vi "Periodic Tasks.vi"(8 "error in":errorcluster) -> ()   [LabVIEW 2019]
doc: "This VI runs in parallel to other tasks. It can contain as many user-defined periodic loops as you need. These can carry out PID or other sorts of timed response."
uses:
  <vilib>/Rock Robotics/WPI/ThirdParty/Sensors/navX/_TypeDefs/Flags/Z900_navX_Flags_HardwareRevTypeDef.ctl
  <vilib>/Rock Robotics/WPI/ThirdParty/Sensors/navX/_TypeDefs/Flags/Z900_navX_Flags_OmnimountConfigTypeDef.ctl
  <vilib>/Rock Robotics/WPI/ThirdParty/Sensors/navX/_TypeDefs/Flags/Z900_navX_Flags_OpStatusTypeDef.ctl
  <vilib>/Rock Robotics/WPI/ThirdParty/Sensors/navX/_TypeDefs/Flags/Z900_navX_Flags_CalibrationStatusTypeDef.ctl
  <vilib>/Rock Robotics/WPI/ThirdParty/Sensors/navX/_TypeDefs/Z900_navX_SerialStreamTypeDef.ctl
  <vilib>/Rock Robotics/WPI/ThirdParty/Sensors/navX/_TypeDefs/FRIC_navX_TestStatesTypeDef_I2C.ctl
  <vilib>/Rock Robotics/WPI/ThirdParty/Sensors/navX/_TypeDefs/FRIC_navX_DeviceNumbersTypeDef.ctl
  <vilib>/Rock Robotics/WPI/Utilities/WPI_GetSetVariantRefNum.vi
  <vilib>/Rock Robotics/Network Tables/NT Write Number.vi
  <vilib>/Rock Robotics/Network Tables/NT Read Number.vi
  <vilib>/Rock Robotics/WPI/ThirdParty/Sensors/navX/_Processing Loop/FRIC_navX_Internal_SPI_ProcessingLoop.vi
  <vilib>/Rock Robotics/WPI/ThirdParty/Sensors/navX/_Processing Loop/FRIC_navX_Internal_I2C_ProcessingLoop.vi
  <vilib>/Rock Robotics/WPI/ThirdParty/Sensors/navX/_Processing Loop/FRIC_navX_Internal_Serial_ProcessingLoop.vi
  <vilib>/Rock Robotics/WPI/ThirdParty/Sensors/navX/_Processing Loop/FRIC_navX_Internal_USB_ProcessingLoop.vi
panel:
  in  "Tab Control":enum32{"Device 0", "Device 1"}(tab)
  out "String":string
  in  "Next":bool
  in  "Exit":bool
  out "Warning":bool
  in  "Change Serial Stream":bool
  out "Connected":bool
  out "Displacement":T1 {"Velocity X" format="%.8f"; "Velocity Y" format="%.8f"; "Velocity Z" format="%.8f"; "Displace X" format="%.8f"; "Displace Y" format="%.8f"; "Displace Z" format="%.8f"}
  out "MPUTemp":dbl format="%.2f"
  out "Board Information":T4 {"Board"."Hardware Revision" items=["navX-MXP"=33, "navX-Micro"=40]; "Omnimount Config" items=["DEFAULT", "X_UP", "X_DOWN", "Y_UP", "Y_DOWN", "Z_UP", "Z_DOWN"]}
  out "Linear Acceleration":cluster{"X":dbl, "Y":dbl, "Z":dbl} {"X" format="%.6f"; "Y" format="%.6f"; "Z" format="%.6f"}
  out "Quaternion":T5 {"Quat W" format="%.8f"; "Quat X" format="%.8f"; "Quat Y" format="%.8f"; "Quat Z" format="%.8f"}
  out "Status":T8 {"OP Status" items=["INITIALIZING", "SELFTEST_IN_PROGRESS", "ERROR", "IMU_AUTOCAL_IN_PROGRESS", "NORMAL"]; "Calibration Status" items=["IMU_CAL_STATE_MASK"=3, "IMU_CAL_STATE_INPROGRESS"=0, "IMU_CAL_STATE_ACCUMULATE"=1, "IMU_CAL_STATE_COMPLETE"=2]}
  out "YRPHfH":T9 {"Yaw" format="%.2f"; "Roll" format="%.2f"; "Pitch" format="%.2f"; "Heading" format="%.2f"; "Fused Heading" format="%.2f"}
  out "Timestamp":u32
  out "Error":bool
  out "error":errorcluster
  in  "Zero Yaw":bool
  in  "Zero Displacement":bool
  in  "Zero Velocity":bool
  out "Raw Values":T10 {"Accel X" format="%.8f"; "Accel Y" format="%.8f"; "Accel Z" format="%.8f"; "Gyro X" format="%.8f"; "Gyro Y" format="%.8f"; "Gyro Z" format="%.8f"; "Mag X" format="%.8f"; "Mag Y" format="%.8f"; "Mag Z" format="%.8f"}
  in  "Stream Type":T11=enum."AHRSAndPositioning"
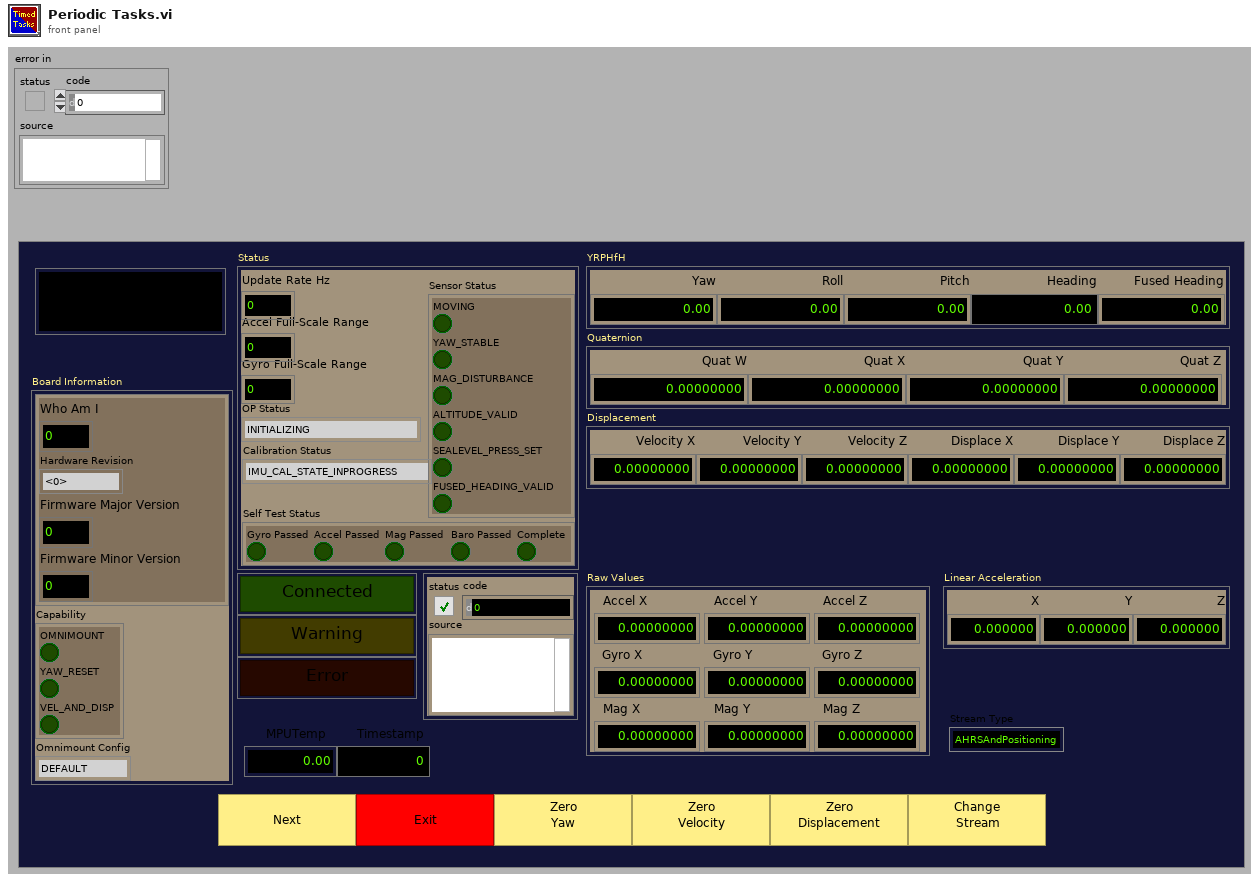
[diagram p1: front panel]
types:
  T1 = cluster{"Velocity X":dbl, "Velocity Y":dbl, "Velocity Z":dbl, "Displace X":dbl, "Displace Y":dbl, "Displace Z":dbl}
  T2 = typedef "Z900_navX_Flags_HardwareRevTypeDef.ctl" = u8
  T3 = typedef "Z900_navX_Flags_OmnimountConfigTypeDef.ctl" = u8
  T4 = cluster{"Board":cluster{"Who Am I":u8, "Hardware Revision":T2, "Firmware Major Version":u8, "Firmware Minor Version":u8}, "Capability":cluster{"OMNIMOUNT":bool, "YAW_RESET":bool, "VEL_AND_DISP":bool}, "Omnimount Config":T3}
  T5 = cluster{"Quat W":dbl, "Quat X":dbl, "Quat Y":dbl, "Quat Z":dbl}
  T6 = typedef "Z900_navX_Flags_OpStatusTypeDef.ctl" = u8
  T7 = typedef "Z900_navX_Flags_CalibrationStatusTypeDef.ctl" = u8
  T8 = cluster{"Update Rate Hz":u8, "Accel Full-Scale Range":u8, "Gyro Full-Scale Range":u16, "OP Status":T6, "Calibration Status":T7, "Sensor Status":cluster{"MOVING":bool, "YAW_STABLE":bool, "MAG_DISTURBANCE":bool, "ALTITUDE_VALID":bool, "SEALEVEL_PRESS_SET":bool, "FUSED_HEADING_VALID":bool}, "Self Test Status":cluster{"Gyro Passed":bool, "Accel Passed":bool, "Mag Passed":bool, "Baro Passed":bool, "Complete":bool}}
  T9 = cluster{"Yaw":dbl, "Roll":dbl, "Pitch":dbl, "Heading":dbl, "Fused Heading":dbl}
  T10 = cluster{"Accel X":dbl, "Accel Y":dbl, "Accel Z":dbl, "Gyro X":dbl, "Gyro Y":dbl, "Gyro Z":dbl, "Mag X":dbl, "Mag Y":dbl, "Mag Z":dbl}
  T11 = typedef "Z900_navX_SerialStreamTypeDef.ctl" = enum16{"YRPH", "Quaterinons", "Gyro/Raw", "AHRS", "AHRSAndPositioning", "AHRSAndPOSTime"}
  T12 = typedef "FRIC_navX_TestStatesTypeDef_I2C.ctl" = enum16{"Unknown", "Start SPI", "Start I2C", "Start Serial", "Start USB", "Hault", "Exit"}
  T13 = typedef "FRIC_navX_DeviceNumbersTypeDef.ctl" = enum16{"Dev0", "Dev1", "Dev2", "Dev3"}
  T14 = cluster{"Velocity X":dbl, "Velocity Y":dbl, "Velocity Z":dbl, "Displacement X":dbl, "Displacement Y":dbl, "Displacement Z":dbl}
  T15 = cluster{"LinearAcceleration X":dbl, "LinearAcceleration Y":dbl, "LinearAcceleration Z":dbl}
  T16 = cluster{"Update Rate Hz":u8, "Accelerometer Full-Scale Range":u8, "Gyro Full-Scale Range":u16, "OP Status":T6, "Calibration Status":T7, "Sensor Status":cluster{"MOVING":bool, "YAW_STABLE":bool, "MAG_DISTURBANCE":bool, "ALTITUDE_VALID":bool, "SEALEVEL_PRESS_SET":bool, "FUSED_HEADING_VALID":bool}, "Self Test Status":cluster{"Gyro Passed":bool, "Accel Passed":bool, "Mag Passed":bool, "Baro Passed":bool, "Complete":bool}}
  T17 = typedef "WPI_JoystickDevRef.ctl" = cluster{"Device":T18}
  T18 = typedef "WPI_JoystickDeviceEnum.ctl" = enum16{"USB 0", "USB 1", "USB 2", "USB 3", "USB 4", "USB 5"}
  T19 = typedef "WPI_RobotDriveDevRef.ctl" = cluster{"DevStatus":errorcluster, "Motors[]":T20[], "Square Inputs":bool, "Max Output":dbl}
  T20 = typedef "WPI_MotorControlDeviceRef.ctl" = cluster{"DeviceStatus":errorcluster, "Type":T21, "PWM":cluster{"PWM Channel":T22, "DeadBand":T23}, "CAN":cluster{"Device Number":u8, "SetOutput VI Ref":variant, "GetOutput VI Ref":variant, "Enable VI Ref":variant, "Disable VI Ref":variant, "Data":variant}, "Invert":bool, "DIO PWM":cluster{"PWM \"Enable\" Channel":T22, "DIOChannel":T24, "PWM Rate":dbl}}
  T21 = typedef "WPI_MotorControlType.ctl" = enum16{"PWM", "CAN", "DIO PWM"}
  T22 = typedef "FPGA_DIOPWMChannel.ctl" = enum8{"PWM 0", "PWM 1", "PWM 2", "PWM 3", "PWM 4", "PWM 5", "PWM 6", "PWM 7", "PWM 8", "PWM 9", "PWM MXP 0", "PWM MXP 1", "PWM MXP 2", "PWM MXP 3", "PWM MXP 4", "PWM MXP 5", "PWM MXP 6", "PWM MXP 7", "PWM MXP 8", "PWM MXP 9", "Invalid"}
  T23 = typedef "WPI_PWMDeadband.ctl" = cluster{"Name":string, "maxPositivePwm":i32, "minPositivePwm":i32, "centerPwm":i32, "maxNegativePwm":i32, "minNegativePwm":i32, "angularRange":u16}
  T24 = typedef "FPGA_DIOChannel.ctl" = enum8{"DIO 0", "DIO 1", "DIO 2", "DIO 3", "DIO 4", "DIO 5", "DIO 6", "DIO 7", "DIO 8", "DIO 9", "DIO MXP 0", "DIO MXP 1", "DIO MXP 2", "DIO MXP 3", "DIO MXP 4", "DIO MXP 5", "DIO MXP 6", "DIO MXP 7", "DIO MXP 8", "DIO MXP 9", "DIO MXP 10", "DIO MXP 11", "DIO MXP 12", "DIO MXP 13", "DIO MXP 14", "DIO MXP 15", "SPI Port CS1", "SPI Port CS2", "SPI Port CS3", "SPI Port MISO", "SPI Port MOSI", "Invalid"}
  T25 = cluster{"JoystickDevRef":T17, "RobotDriveDevRef":T19}
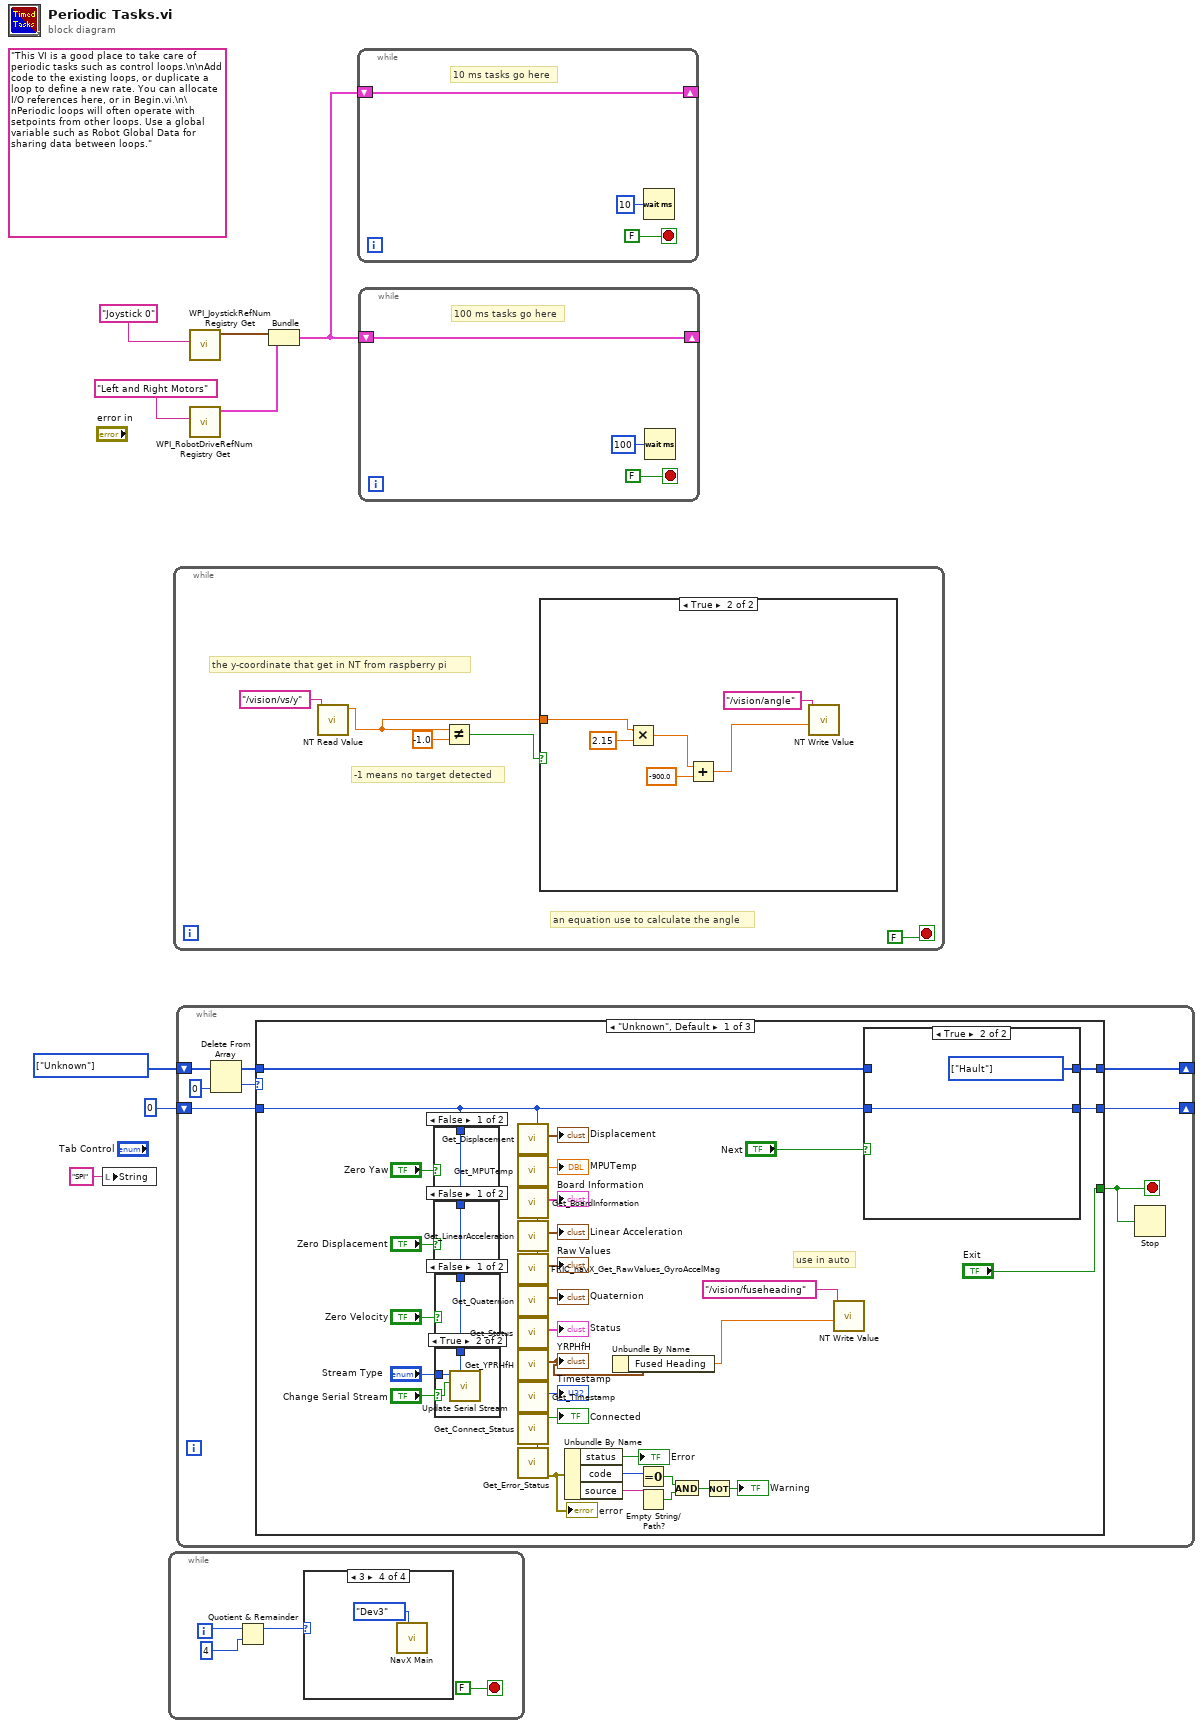
[diagram p0: block diagram]
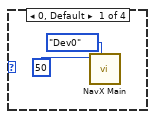
[diagram p2: hidden frame]
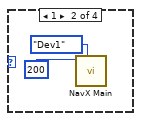
[diagram p3: hidden frame]
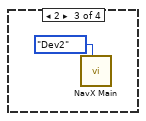
[diagram p4: hidden frame]
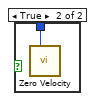
[diagram p7: hidden frame]
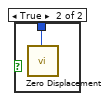
[diagram p8: hidden frame]
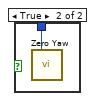
[diagram p9: hidden frame]
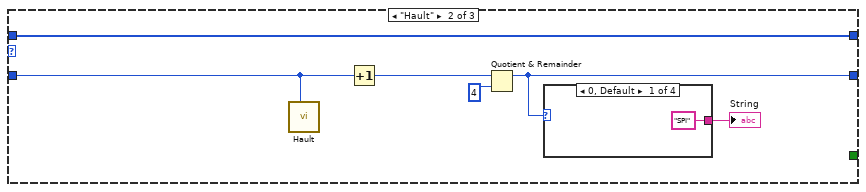
[diagram p10: hidden frame]
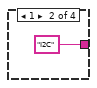
[diagram p11: hidden frame]
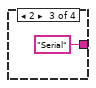
[diagram p12: hidden frame]
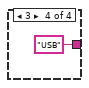
[diagram p13: hidden frame]
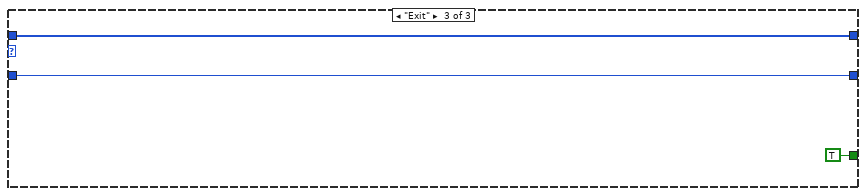
[diagram p14: hidden frame]
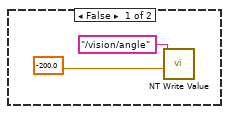
[diagram p15: hidden frame]
diagram:
  w3 = T12[] [enum."Unknown"] items=["Unknown", "Start SPI", "Start I2C", "Start Serial", "Start USB", "Hault", "Exit"]
  (unwired) "This VI is a good place to take care of periodic tasks such as control loops.\n\nAdd code to the existing loops, or duplicate a loop to define a new rate. You can allocate I/O references here, or in Begin.vi.\n\nPeriodic loops will often operate with setpoints from other loops. Use a global variable such as Robot Global Data for sharing data between loops."
  n1 = local write "String"("SPI" ("String")) -> ()
  n2 = while {
    i -> [w9]
    stop <- FALSE stop-if-true
    n3 = Quotient & Remainder(x=w9, y=4 ("x")) -> (x-y*floor(x/y)=w12:i32)  [unwired: 1 out]
    n4 = case shown="3" w12 {
      frame 0, Default {
        n5 = call-poly <vilib>:"NavX Main.vi"("Device Number"=FRIC_navX_DeviceNumbersTypeDef."Dev0", "Rate (4Hz-200Hz)"=50) -> ()  [unwired: 10 in]
      }
      frame 1 {
        n6 = call-poly <vilib>:"NavX Main.vi"("Device Number"=FRIC_navX_DeviceNumbersTypeDef."Dev1", "Rate (4Hz-200Hz)"=200) -> ()  [unwired: 10 in]
      }
      frame 2 {
        n7 = call-poly <vilib>:"NavX Main.vi"("Device Number"=FRIC_navX_DeviceNumbersTypeDef."Dev2") -> ()  [unwired: 11 in]
      }
      frame 3 {
        n8 = call-poly <vilib>:"NavX Main.vi"("Device Number"=FRIC_navX_DeviceNumbersTypeDef."Dev3") -> ()  [unwired: 11 in]
      }
    }
  }
  n9 = while {
    stop <- FALSE stop-if-true
    # "-1 means no target detected"
    # "an equation use to calculate the angle"
    # "the y-coordinate that get in NT from raspberry pi"
    n10 = call-poly <vilib>:"NT Read Value.vi"("Name"="/vision/vs/y") -> ("Numeric"=w21:dbl)  [unwired: 9 in, 1 out]
    n11 = Not Equal?(x=w21, y=-1.0) -> (x != y?=w20:bool)
    n12 = case shown="True" w20 {
      tunnel: w21 -> [_ w30]
      frame False {
        n13 = call-poly <vilib>:"NT Write Value.vi"("Numeric"=-200.0, "Name"="/vision/angle") -> ()  [unwired: 9 in, 1 out]
      }
      frame True {
        n14 = Multiply(x=w30, y=2.15) -> (x*y=w28:dbl)
        n15 = Add(x=w28, y=-900.0) -> (x+y=w26:dbl)
        n16 = call-poly <vilib>:"NT Write Value.vi"("Numeric"=w26, "Name"="/vision/angle") -> ()  [unwired: 9 in, 1 out]
      }
    }
  }
  n17 = while "Scheduling loop" {
    shift-right: [w35] -> _
    shift-left: w3 -> [w39]
    shift-right: [w34] -> _
    shift-left: 0 -> [w33]
    stop <- w32 stop-if-true
    n18 = Delete From Array(array=w39, index=0) -> (deleted portion=w37:T12, array with subset deleted=w36:T12[])  [unwired: 1 in]
    n19 = case shown="\"Unknown\", Default" w37 {
      tunnel: ["Exit" _ TRUE] -> w32
      tunnel: w36 -> [w48 w86 w92]
      tunnel: [w47 w86 w92] -> w35
      tunnel: [w45 w81 w91] -> w34
      tunnel: w33 -> [w44 w83 w91]
      frame "Unknown", Default {
        # "use in auto"
        n20 = case shown="False" "Zero Yaw" {
          tunnel: w44 -> [_ w80]
          frame False {
          }
          frame True {
            n21 = call <vilib>:"Zero Yaw.vi"("Device Number"=w80) -> ()  [unwired: 11 in]
          }
        }
        n22 = case shown="False" "Zero Displacement" {
          tunnel: w44 -> [_ w79]
          frame False {
          }
          frame True {
            n23 = call <vilib>:"Zero Displacement.vi"("Device Number"=w79) -> ()  [unwired: 11 in]
          }
        }
        n24 = case shown="False" "Zero Velocity" {
          tunnel: w44 -> [_ w78]
          frame False {
          }
          frame True {
            n25 = call <vilib>:"Zero Velocity.vi"("Device Number"=w78) -> ()  [unwired: 11 in]
          }
        }
        n26 = case shown="True" "Change Serial Stream" {
          selector: "Change Serial Stream" -> [_ w75]
          tunnel: w44 -> [_ w77]
          tunnel: "Stream Type" -> [_ w76]
          frame False {
          }
          frame True {
            n27 = call <vilib>:"Update Serial Stream.vi"("Device Number"=w77, "Update"=w75, "Stream Type"=w76) -> ()  [unwired: 9 in]
          }
        }
        n28 = call <vilib>:"Get_Displacement.vi"("Device Number"=w44) -> ("Displacement"=→"Displacement":T14)  [unwired: 10 in]
        n29 = call <vilib>:"Get_MPUTemp.vi"("Device Number"=w44) -> ("MPUTemp"=→"MPUTemp":dbl)  [unwired: 10 in]
        n30 = call <vilib>:"Get_BoardInformation.vi"("Device Number"=w44) -> ("Board Information"=→"Board Information":T4)  [unwired: 10 in]
        n31 = call <vilib>:"Get_LinearAcceleration.vi"("Device Number"=w44) -> ("Linear Acceleration"=→"Linear Acceleration":T15)  [unwired: 10 in]
        n32 = call <vilib>:"FRIC_navX_Get_RawValues_GyroAccelMag.vi"("Device Number"=w44) -> ("Raw Values (out)"=→"Raw Values":T10)  [unwired: 10 in]
        n33 = call <vilib>:"Get_Quaternion.vi"("Device Number"=w44) -> ("Quaternion"=→"Quaternion":T5)  [unwired: 10 in]
        n34 = call <vilib>:"Get_Status.vi"("Device Number"=w44) -> ("Status"=→"Status":T16)  [unwired: 10 in]
        n35 = call <vilib>:"Get_YPRHfH.vi"("Device Number"=w44) -> ("YRPHfH"=w42:T9)  [unwired: 10 in]
        "YRPHfH" <- w42
        n36 = call <vilib>:"Get_Timestamp.vi"("Device Number"=w44) -> ("Timestamp"=→"Timestamp":u32)  [unwired: 10 in]
        n37 = call <vilib>:"Get_Connect_Status.vi"("Device Number"=w44) -> ("Connected"=→"Connected":bool)  [unwired: 10 in]
        n38 = call <vilib>:"Get_Error_Status.vi"("Device Number"=w44) -> ("error out"=w63:errorcluster)  [unwired: 10 in]
        "error" <- w63
        n39 = Unbundle By Name(w63) -> ("status"=→"Error":bool, "code"=w65:i32, "source"=w66:string)
        n40 = Unbundle By Name(w42) -> ("Fused Heading"=w40:dbl)
        n41 = Equal To 0?(x=w65) -> (x = 0?=w67:bool)
        n42 = Empty String/Path?(string/path=w66) -> (empty?=w68:bool)
        n43 = And(x=w67, y=w68) -> (x .and. y?=w69:bool)
        n44 = Not(x=w69) -> (.not. x?=→"Warning":bool)
        n45 = call-poly <vilib>:"NT Write Value.vi"("Numeric"=w40, "Name"="/vision/fuseheading") -> ()  [unwired: 9 in, 1 out]
        n46 = case shown="True" "Next" {
          tunnel: w48 -> [w72 _]
          tunnel: [w72 w73] -> w47
          tunnel: [w71 w74] -> w45
          tunnel: w44 -> [w71 w74]
          frame False {
          }
          frame True {
            w73 = T12[] [enum."Hault"] items=["Unknown", "Start SPI", "Start I2C", "Start Serial", "Start USB", "Hault", "Exit"]
          }
        }
      }
      frame "Hault" {
        n47 = call <vilib>:"Hault.vi"("Device Number"=w83) -> ()  [unwired: 11 in]
        n48 = Increment(x=w83) -> (x+1=w85:i32)
        n49 = Quotient & Remainder(x=w85, y=4) -> (x-y*floor(x/y)=w81:i32)  [unwired: 1 out]
        n50 = case shown="0, Default" w81 {
          tunnel: ["SPI" ("String") "I2C" ("String") "Serial" ("String") "USB" ("String")] -> w82
          frame 0, Default {
          }
          frame 1 {
          }
          frame 2 {
          }
          frame 3 {
          }
        }
        "String" <- w82
      }
      frame "Exit" {
      }
    }
    n51 = Stop(stop? (T)=w32) -> ()
  }
  n52 = call <vilib>:"WPI_JoystickRefNum Registry Get.vi"("refnum name"="Joystick 0") -> ("JoystickDevRef"=w6:T17)  [unwired: 1 in, 9 out]
  n53 = call <vilib>:"WPI_RobotDriveRefNum Registry Get.vi"("refnum name"="Left and Right Motors") -> ("RobotDriveDevRef"=w5:T19)  [unwired: 1 in, 9 out]
  n54 = Bundle("JoystickDevRef"=w6, "RobotDriveDevRef"=w5) -> (w4:T25)  [unwired: 1 out]
  n55 = while {
    shift-right: [w94] -> _
    shift-left: w4 -> [w94]
    stop <- FALSE stop-if-true
    # "10 ms tasks go here"
    n56 = Wait (ms)(milliseconds to wait=u32 10) -> ()  [unwired: 1 out]
  }
  n57 = while {
    shift-right: [w97] -> _
    shift-left: w4 -> [w97]
    stop <- FALSE stop-if-true
    # "100 ms tasks go here"
    n58 = Wait (ms)(milliseconds to wait=u32 100) -> ()  [unwired: 1 out]
  }
